vi "line to strings.vi"(11 "line":T1) -> (3 "strings":string[](array[string]))   [LabVIEW 2013, in "CVT editor node.lvclass"]
uses:
  CVT editor node.lvclass
  table line.ctl
  <vilib>/NI/Tag Bus Module Framework/channel/TBM channel.lvclass
  <vilib>/NI/Tag Bus/tag/tag descriptor.lvclass/tag descriptor.ctl
  <vilib>/NI/Tag Bus Module Framework/channel/TBM channel.lvclass/TBM channel.ctl
  <vilib>/NI/Tag Bus/tag/read tag name.vi
  <vilib>/NI/Tag Bus Module Framework/channel/Read channel classification.vi
  <vilib>/NI/Tag Bus/tag/read data type.vi
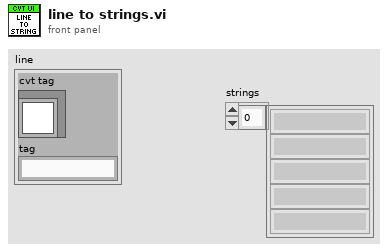
[diagram p1: front panel]
types:
  T1 = typedef "CVT editor node.lvclass/table line.ctl" = cluster{"cvt tag":refnum<class "TBM channel.lvclass">, "tag":string}
  T2 = typedef "TBM channel.lvclass/channel classification.ctl" = enum16{"input data", "output data", "processing parameter", "processing result"}
  T3 = typedef "tag bus.lvlib/tag descriptor.lvclass/Data Type.ctl" = enum16{"Double", "Single", "I64", "I32", "I16", "I8", "U64", "U32", "U16", "U8", "Boolean", "String", "Array of Double", "Array of Single", "Array of I64", "Array of I32", "Array of I16", "Array of I8", "Array of U64", "Array of U32", "Array of U16", "Array of U8", "Array of Boolean", "Array of String"}
  T4 = typedef "CVT editor node.lvclass/permissions.ctl" = enum16{"Read from CVT", "Write to CVT"}
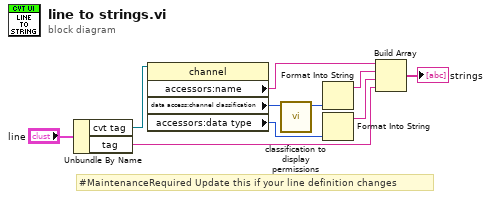
[diagram p0: block diagram]
diagram:
  # "#MaintenanceRequired Update this if your line definition changes"
  n1 = Unbundle By Name("line") -> ("cvt tag"=w4:refnum<class "TBM channel.lvclass">, "tag"=w8:string)
  n2 = property class="channel"(reference=w4) -> ("accessors:name"=w1:string, "data access:channel classification"=w3:T2, "accessors:data type"=w2:T3)  [unwired: 1 in, 2 out]
  n3 = call "classification to display permissions.vi"("channel classification"=w3) -> ("permissions"=w6:T4)  [unwired: 10 in]
  n4 = Format Into String(w6) -> (resulting string=w5:string)  [unwired: 3 in, 1 out]
  n5 = Format Into String(w2) -> (resulting string=w9:string)  [unwired: 3 in, 1 out]
  n6 = Build Array(w1, w5, w9, w8) -> (→"strings":string[])
